vi "Configure Event Search Characteristic.vi"(8 "error in (no error)":errorcluster, 9 "Event Search Type (0: Edge)":i32(ring) items=["Edge", "Glitch", "Runt", "Transition", "Serial 1", "Serial 2", "Peak"], 10 "Enable Event Search (F: Disable)":bool, 11 "VISA resource name":refnum<visa-resource-name>) -> (0 "error out":errorcluster, 3 "VISA resource name out":refnum<visa-resource-name>)   [LabVIEW 2017, in "Agilent 2000 3000 X-Series.lvlib"]
doc: "Configures the basic function of event search.\n\nNotes:\nThis VI is not supported by EDUX1052A/G, DSOX1202A/G, DSOX1204A/G models."
uses:
  Agilent 2000 3000 X-Series.lvlib
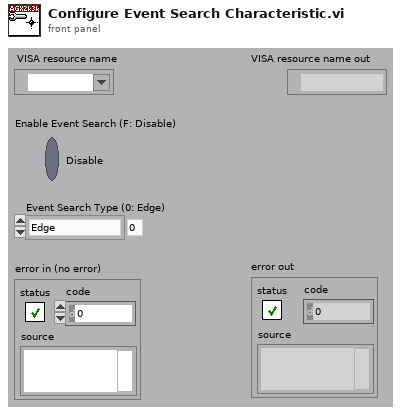
[diagram p1: front panel]
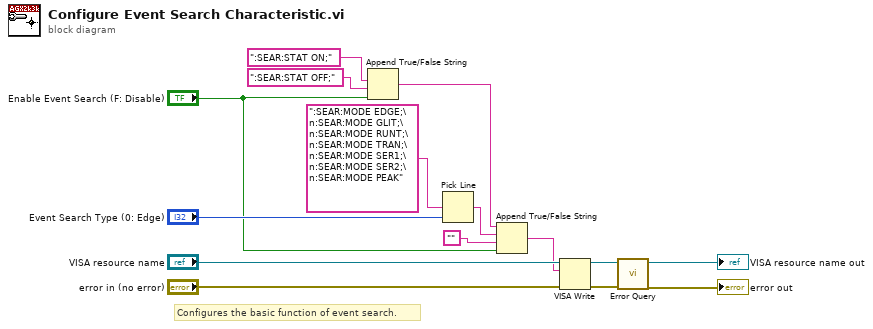
[diagram p0: block diagram]
diagram:
  # "Configures the basic function of event search."
  n1 = Append True/False String(1:"Enable Event Search (F: Disable)", 2:":SEAR:STAT OFF;", 3:":SEAR:STAT ON;") -> (0:w4:string)  [unwired: 1 out]
  n2 = Pick Line(multi-line string=":SEAR:MODE EDGE;\n:SEAR:MODE GLIT;\n:SEAR:MODE RUNT;\n:SEAR:MODE TRAN;\n:SEAR:MODE SER1;\n:SEAR:MODE SER2;\n:SEAR:MODE PEAK", line index="Event Search Type (0: Edge)") -> (output string=w3:string)  [unwired: 1 out]
  n3 = Append True/False String(1:"Enable Event Search (F: Disable)", 2:"", 3:w3, 4:w4) -> (0:w2:string)
  n4 = VISA Write(VISA resource name="VISA resource name", write buffer=w2, error in (no error)="error in (no error)") -> (VISA resource name out=w9:refnum<visa-resource-name>, error out=w8:errorcluster)  [unwired: 1 out]
  n5 = call "Error Query.vi"("error in (no error)"=w8, "VISA resource name"=w9) -> ("error out"=→"error out":errorcluster, "VISA resource name out"=→"VISA resource name out":refnum<visa-resource-name>)  [unwired: 8 out]
